vi "main_loop.vi"(8 "error in (no error)":errorcluster, 11 "control references":T2) -> (0 "error out":errorcluster)   [LabVIEW 2010]
uses:
  type_definitions/clusters/controls_refs.ctl
  type_definitions/enumerations/state_enumeration.ctl
  type_definitions/enumerations/main_trigger_enum.ctl
  type_definitions/clusters/state_data_cluster.ctl
  type_definitions/clusters/top_level_config_cluster.ctl
  common/clusters/plugin_specification.ctl
  common/enumerations/top-level_component_type_enum.ctl
  common/classes/GenericComponent/GenericComponent/GenericComponent.lvclass
  type_definitions/enumerations/main_control_types.ctl
  common/classes/NoteBook/Notebook/Notebook.lvclass
panel:
  out "state":T1
  out "Main statechart loop counter":i32
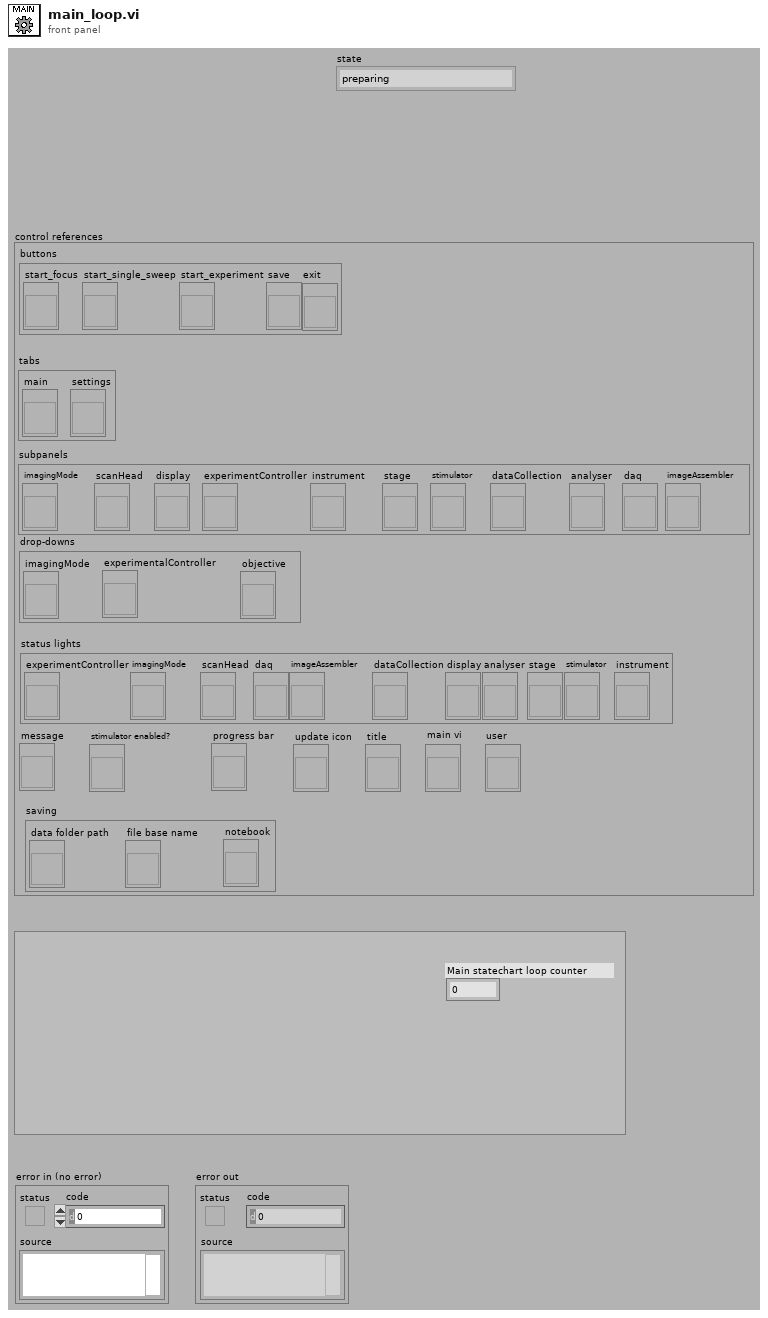
[diagram p1: front panel]
types:
  T1 = typedef "state_enumeration.ctl" = enum16{"preparing", "ready", "saving"}
  T2 = typedef "controls_refs.ctl" = cluster{"buttons":cluster{"start_focus":refnum<vi>, "start_single_sweep":refnum<vi>, "start_experiment":refnum<vi>, "save":refnum<vi>, "exit":refnum<vi>}, "tabs":cluster{"main":refnum<vi>, "settings":refnum<vi>}, "subpanels":cluster{"imagingMode":refnum<vi>, "scanHead":refnum<vi>, "display":refnum<vi>, "experimentController":refnum<vi>, "instrument":refnum<vi>, "stage":refnum<vi>, "stimulator":refnum<vi>, "dataCollection":refnum<vi>, "analyser":refnum<vi>, "daq":refnum<vi>, "imageAssembler":refnum<vi>}, "drop-downs":cluster{"imagingMode":refnum<vi>, "experimentalController":refnum<vi>, "objective":refnum<vi>}, "status lights":cluster{"experimentController":refnum<vi>, "imagingMode":refnum<vi>, "scanHead":refnum<vi>, "daq":refnum<vi>, "imageAssembler":refnum<vi>, "dataCollection":refnum<vi>, "display":refnum<vi>, "analyser":refnum<vi>, "stage":refnum<vi>, "stimulator":refnum<vi>, "instrument":refnum<vi>}, "message":refnum<vi>, "stimulator enabled?":refnum<vi>, "saving":cluster{"data folder path":refnum<vi>, "file base name":refnum<vi>, "notebook":refnum<vi>}, "progress bar":refnum<vi>, "update icon":refnum<vi>, "title":refnum<vi>, "main vi":refnum<vi>, "user":refnum<vi>}
  T3 = typedef "main_trigger_enum.ctl" = enum16{"NULL", "initialise", "terminate", "start", "stop", "change objective", "change experimentController", "change imagingMode", "save notebook", "started saving", "finished saving", "expCtr ready", "expCtr missing", "imgMd ready", "imgMd missing", "scanHd ready", "scanHd missing", "DAQ ready", "DAQ missing", "imgAsm ready", "imgAsm missing", "dataColl ready", "dataColl missing", "display ready", "display missing", "analysr ready", "analysr missing", "instrmnt ready", "instrmnt missing", "stimltr ready", "stimltr missing", "stage ready", "stage missing"}
  T4 = typedef "state_data_cluster.ctl" = cluster{"configuration":T5, "previous message display parameters":cluster{"previous  string":string, "BG slider":u32, "previously visible?":bool}}
  T5 = typedef "top_level_config_cluster.ctl" = cluster{"experimentControllers":T6[], "default experimentController":string, "imagingModes":T6[], "default imagingMode":string, "stage":T6, "objectives":T6[], "default objective":string}
  T6 = typedef "plugin_specification.ctl" = cluster{"class path":string, "configuration":string, "label":string, "settings name":string}
  T7 = typedef "top-level_component_type_enum.ctl" = enum16{"undefined", "ImagingMode", "ScanHead", "DAQ", "ImageAssembler", "Display", "DataCollection", "Analyser", "Stimulator", "ExperimentController", "Instrument", "Stage"}
  T8 = enum8{"Enabled", "Disabled", "Disabled and Grayed Out"}
  T9 = cluster{"previous  string":string, "BG slider":u32, "previously visible?":bool}
  T10 = typedef "main_control_types.ctl" = enum16{"scan start button", "experimentController subpanel", "imagingMode subpanel", "scanHead subpanel", "dataCollection subpanel", "display subpanel", "analyser subpanel", "stimulator subpanel", "imagingMode drop-down", "experimentController drop-down", "objective drop-down", "exit button"}
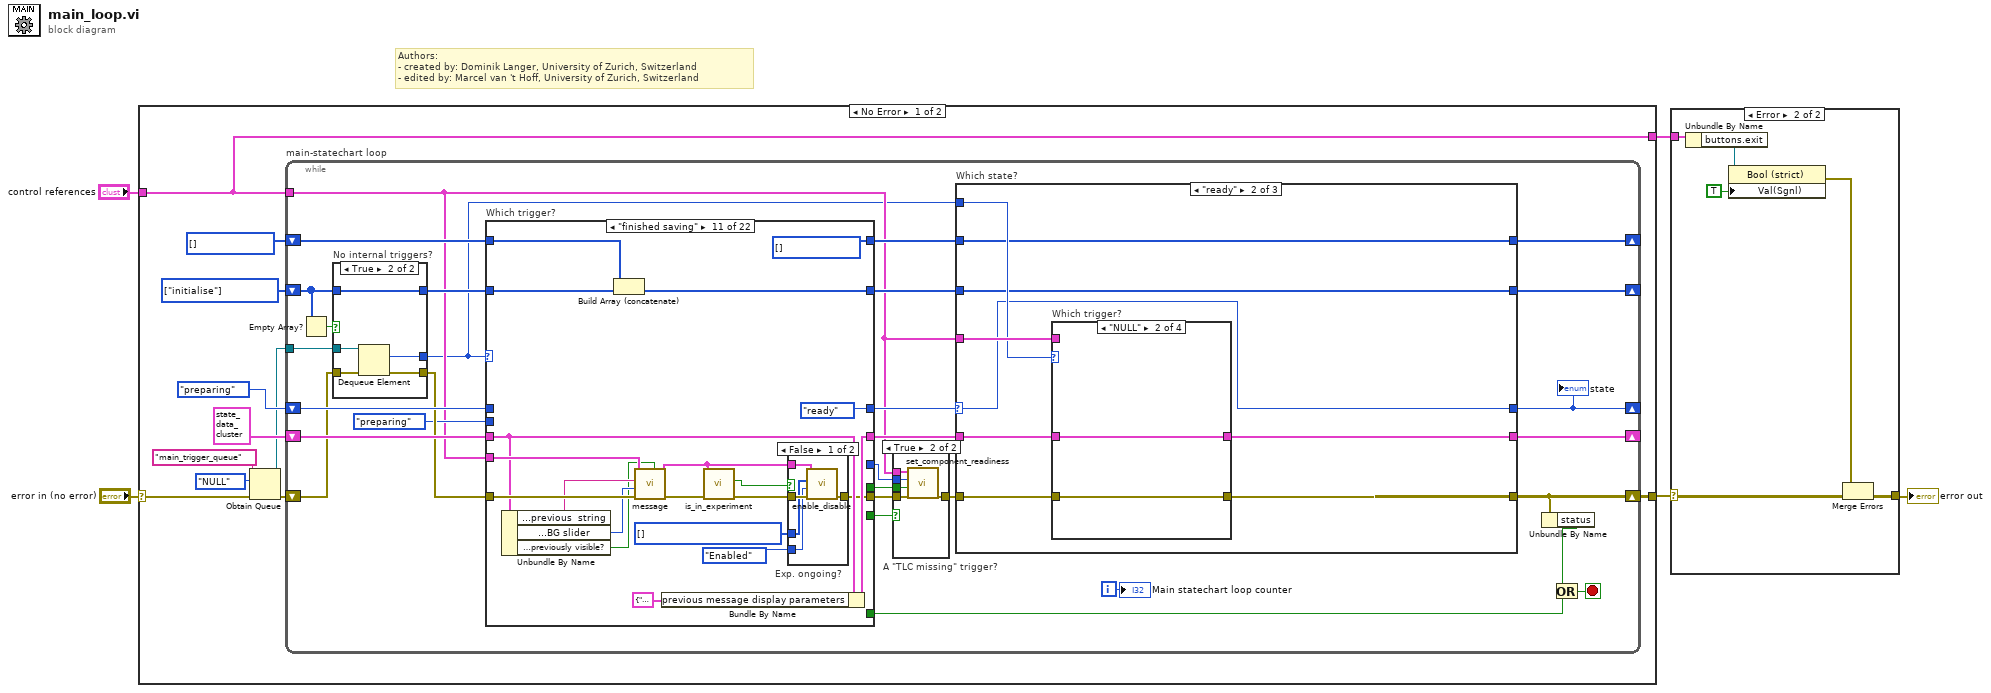
[diagram p0: block diagram]
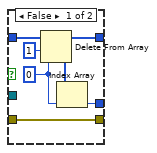
[diagram p3: hidden frame]
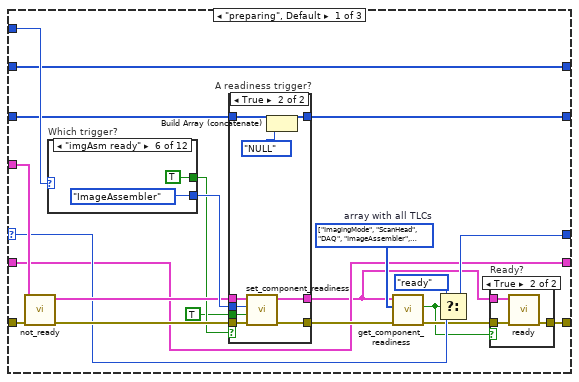
[diagram p5: hidden frame]
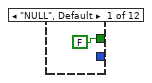
[diagram p8: hidden frame]
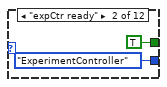
[diagram p9: hidden frame]
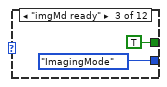
[diagram p10: hidden frame]
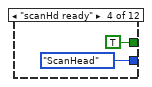
[diagram p11: hidden frame]
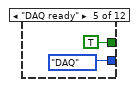
[diagram p12: hidden frame]
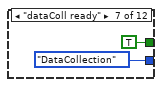
[diagram p13: hidden frame]
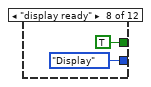
[diagram p14: hidden frame]
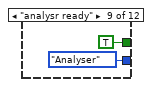
[diagram p15: hidden frame]
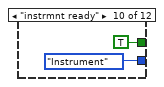
[diagram p16: hidden frame]
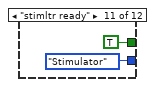
[diagram p17: hidden frame]
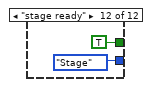
[diagram p18: hidden frame]
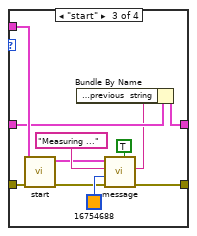
[diagram p20: hidden frame]
diagram:
  # "Authors: \n- created by: Dominik Langer, University of Zurich, Switzerland\n- edited by: Marcel van 't Hoff, University of Zurich, Switzerland"
  n1 = case shown="No Error" "error in (no error)" {
    selector: "error in (no error)" -> [w11 w376]
    tunnel: [w16 w376] -> w3
    tunnel: "control references" -> [w15 w375]
    tunnel: [w15 w375] -> w1
    frame No Error {
      w6 = T3[] [] items=["NULL", "initialise", "terminate", "start", "stop", "change objective", "change experimentController", "change imagingMode", "save notebook", "started saving", "finished saving", "expCtr ready", "expCtr missing", "imgMd ready", "imgMd missing", "scanHd ready", "scanHd missing", "DAQ ready", "DAQ missing", "imgAsm ready", "imgAsm missing", "dataColl ready", "dataColl missing", "display ready", "display missing", "analysr ready", "analysr missing", "instrmnt ready", "instrmnt missing", "stimltr ready", "stimltr missing", "stage ready", "stage missing"]
      w12 = T3[] [enum."initialise"] items=["NULL", "initialise", "terminate", "start", "stop", "change objective", "change experimentController", "change imagingMode", "save notebook", "started saving", "finished saving", "expCtr ready", "expCtr missing", "imgMd ready", "imgMd missing", "scanHd ready", "scanHd missing", "DAQ ready", "DAQ missing", "imgAsm ready", "imgAsm missing", "dataColl ready", "dataColl missing", "display ready", "display missing", "analysr ready", "analysr missing", "instrmnt ready", "instrmnt missing", "stimltr ready", "stimltr missing", "stage ready", "stage missing"]
      n2 = Obtain Queue(name (unnamed)="main_trigger_queue", element data type=main_trigger_enum."NULL" ("main trigger"), error in (no error)=w11) -> (queue out=w7:refnum<queue>, error out=w10:errorcluster)  [unwired: 2 in, 1 out]
      n3 = while "main-statechart loop" {
        tunnel: w15 -> [w19]
        shift-right: [w36] -> w16
        shift-left: w10 -> [w27]
        shift-right: [w37] -> _
        shift-left: T4 {"configuration"={"experimentControllers"=[], "default experimentController"="", "imagingModes"=[], "default imagingMode"="", "stage"={"class path"="", "configuration"="", "label"="", "settings name"=""}, "objectives"=[], "default objective"=""}, "previous message display parameters"={"previous  string"="", "BG slider"=16754688, "previously visible?"=FALSE}} ("state data") -> [w42]
        shift-right: [w39] -> _
        shift-left: state_enumeration."preparing" ("state enumeration") -> [w41]
        shift-right: [w35] -> _
        shift-left: w12 -> [w30]
        tunnel: w7 -> [w28]
        shift-right: [w24] -> _
        shift-left: w6 -> [w21]
        i -> [w46]
        stop <- w45 stop-if-true
        n4 = Empty Array?(array=w30) -> (empty?=w29:bool)
        n5 = case "No internal triggers?" shown="True" w29 {
          tunnel: w30 -> [w53 w58]
          tunnel: [w52 w58] -> w23
          tunnel: [w48 w56] -> w18
          tunnel: w28 -> [_ w57]
          tunnel: w27 -> [w47 w55]
          tunnel: [w47 w54] -> w26
          frame False {
            w49 = 0 ("index")
            n6 = Delete From Array(array=w53, length=1, index=w49) -> (deleted portion=w51:T3[], array with subset deleted=w52:T3[])
            n7 = Index Array(array=w51, index=w49) -> (element=w48:T3)
          }
          frame True {
            n8 = Dequeue Element(queue=w57, error in (no error)=w55) -> (element=w56:T3, error out=w54:errorcluster)  [unwired: 1 in, 2 out]
          }
        }
        n9 = case "Which trigger?" shown="\"finished saving\"" w18 {
          tunnel: w26 -> [w176 w185 w191 w202 w207 w216 w224 w233 w239 w246 w289 w303 w311 w318 w325 w332 w339 w346 w353 w360 w367 w374]
          tunnel: w19 -> [_ w186 w193 _ _ w214 w220 w231 _ w244 w288 _ _ _ _ _ _ _ _ _ _ _]
          tunnel: [w176 w184 w194 w202 w207 w215 w223 w232 w238 w258 w281 w303 w311 w318 w325 w332 w339 w346 w353 w360 w367 w374] -> w33
          tunnel: [_ _ TRUE _ _ _ _ _ _ _ _ _ _ _ _ _ _ _ _ _ _ _] -> w44
          tunnel: w42 -> [w177 w183 w196 w201 w206 w212 w221 w229 w237 w251 w283 w304 w310 w317 w324 w331 w338 w345 w352 w359 w366 w373]
          tunnel: [w177 w181 w196 w201 w206 w212 w221 w229 w237 w255 w282 w304 w310 w317 w324 w331 w338 w345 w352 w359 w366 w373] -> w38
          tunnel: w41 -> [w175 w180 _ w200 w205 w210 w219 w227 w236 _ _ _ _ _ _ _ _ _ _ _ _ _]
          tunnel: [w175 w180 state_enumeration."preparing" ("state enumeration") w200 w205 w210 w219 w227 w236 state_enumeration."saving" ("state enumeration") state_enumeration."ready" ("state enumeration") w299 w307 w314 w321 w328 w335 w342 w349 w356 w363 w370] -> w40
          tunnel: [_ _ _ _ _ _ _ _ _ _ _ top-level_component_type_enum."ExperimentController" ("top-level component type") top-level_component_type_enum."ImagingMode" ("top-level component type") top-level_component_type_enum."ScanHead" ("top-level component type") top-level_component_type_enum."DAQ" ("top-level component type") top-level_component_type_enum."ImageAssembler" ("top-level component type") top-level_component_type_enum."DataCollection" ("top-level component type") top-level_component_type_enum."Display" ("top-level component type") top-level_component_type_enum."Analyser" ("top-level component type") top-level_component_type_enum."Instrument" ("top-level component type") top-level_component_type_enum."Stimulator" ("top-level component type") top-level_component_type_enum."Stage" ("top-level component type")] -> w17
          tunnel: [_ _ _ _ _ _ _ _ _ _ _ FALSE _ _ _ _ _ _ _ _ _ _] -> w32
          tunnel: [_ _ _ _ _ _ _ _ _ _ _ TRUE TRUE TRUE TRUE TRUE TRUE TRUE TRUE TRUE TRUE TRUE] -> w31
          tunnel: state_enumeration."preparing" ("state enumeration") -> [_ _ _ _ _ _ _ _ _ _ _ w299 w307 w314 w321 w328 w335 w342 w349 w356 w363 w370]
          tunnel: w21 -> [w174 w179 w188 w199 w204 w209 w218 w226 w235 w248 w278 w298 w306 w313 w320 w327 w334 w341 w348 w355 w362 w369]
          tunnel: w23 -> [w173 w178 w187 w198 w203 w208 w217 w225 w234 w247 w277 w297 w305 w312 w319 w326 w333 w340 w347 w354 w361 w368]
          tunnel: [w173 w178 w187 w198 w203 w208 w217 w225 w234 w247 w276 w297 w305 w312 w319 w326 w333 w340 w347 w354 w361 w368] -> w22
          tunnel: [w174 w179 w188 w199 w204 w209 w218 w226 w235 w248 w275 w298 w306 w313 w320 w327 w334 w341 w348 w355 w362 w369] -> w20
          frame "NULL", Default {
          }
          frame "initialise" {
            n10 = call "initialise_main.vi"("error in (no error)"=w185, "control references in"=w186) -> ("error out"=w184:errorcluster, "configuration"=w182:T5)  [unwired: 8 in]
            n11 = Bundle By Name(cluster=w183, "configuration"=w182) -> (w181:T4)
          }
          frame "terminate" {
            n12 = Unbundle By Name(w193) -> ("buttons.exit"=w192:refnum<vi>)
            n13 = property class="Bool (strict)"(reference=w192, error in=w191, "Val(Sgnl)"=TRUE ("Value (Signaling)")) -> (error out=w190:errorcluster)  [unwired: 1 out]
            n14 = call "terminate_main.vi"("error in (no error)"=w190) -> ("error out"=w194:errorcluster)  [unwired: 10 in]
          }
          frame "start" {
          }
          frame "stop" {
          }
          frame "change objective" {
            n15 = Unbundle By Name(w212) -> ("configuration.objectives"=w211:T6[])
            n16 = Unbundle By Name(w214) -> ("drop-downs.objective"=w213:refnum<vi>)
            n17 = call "change_objective.vi"("error in (no error)"=w216, "objectives"=w211, "objective"=w213) -> ("error out"=w215:errorcluster)  [unwired: 8 in]
          }
          frame "change experimentController" {
            n18 = Unbundle By Name(w221) -> ("configuration.experimentControllers"=w222:T6[])
            n19 = call "change_experimentController.vi"("error in (no error)"=w224, "experimentControllers"=w222, "control references in"=w220) -> ("error out"=w223:errorcluster)  [unwired: 8 in]
          }
          frame "change imagingMode" {
            n20 = Unbundle By Name(w229) -> ("configuration.imagingModes"=w228:T6[])
            n21 = Unbundle By Name(w231) -> ("drop-downs.imagingMode"=w230:refnum<vi>)
            n22 = call "change_imagingMode.vi"("error in (no error)"=w233, "imagingModes"=w228, "imagingMode"=w230) -> ("error out"=w232:errorcluster)  [unwired: 8 in]
          }
          frame "save notebook" {
            n23 = call-dynamic "get_notebook.vi"("error in (no error)"=w239, "GenericComponent in"=refnum<class "GenericComponent.lvclass"> refnum) -> ("error out"=w240:errorcluster, "notebook"=w241:refnum<class "Notebook.lvclass">)  [unwired: 7 in, 1 out]
            n24 = call "save.vi"("error in (no error)"=w240, "Notebook in"=w241) -> ("error out"=w238:errorcluster)  [unwired: 8 in, 1 out]
          }
          frame "started saving" {
            w256 = T10[] [] items=["scan start button", "experimentController subpanel", "imagingMode subpanel", "scanHead subpanel", "dataCollection subpanel", "display subpanel", "analyser subpanel", "stimulator subpanel", "imagingMode drop-down", "experimentController drop-down", "objective drop-down", "exit button"] ("controls")
            n25 = call "is_in_experiment.vi"("error in (no error)"=w246, "control references"=w244) -> ("error out"=w245:errorcluster, "in experiment?"=w243:bool)  [unwired: 8 in]
            n26 = case "Experiment ongoing?" shown="False" w243 {
              tunnel: w245 -> [w268 w270]
              tunnel: [w267 w270] -> w261
              tunnel: w244 -> [w266 w269]
              tunnel: T8."Disabled and Grayed Out" ("state") -> [w265 _]
              tunnel: w256 -> [w264 _]
              tunnel: [w263 w269] -> w250
              frame False {
                n27 = call "enable_disable.vi"("error in (no error)"=w268, "state"=w265, "controls"=w264, "control references in"=w266) -> ("error out"=w267:errorcluster, "control references out"=w263:T2)  [unwired: 6 in]
              }
              frame True {
              }
            }
            n28 = call "message.vi"("visible?"=TRUE, "error in (no error)"=w261, "BG slider"=u32 16751378, "text"="Saving ...", "control references in"=w250) -> ("error out"=w258:errorcluster, "previous text"=w254:string, "previously visible?"=w252:bool, "previous BG colour"=w253:u32)  [unwired: 2 in, 1 out]
            n29 = Bundle By Name(cluster=w251, "previous message display parameters.previous  string"=w254, "previous message display parameters.BG slider"=w253, "previous message display parameters.previously visible?"=w252) -> (w255:T4)
          }
          frame "finished saving" {
            w275 = T3[] [] items=["NULL", "initialise", "terminate", "start", "stop", "change objective", "change experimentController", "change imagingMode", "save notebook", "started saving", "finished saving", "expCtr ready", "expCtr missing", "imgMd ready", "imgMd missing", "scanHd ready", "scanHd missing", "DAQ ready", "DAQ missing", "imgAsm ready", "imgAsm missing", "dataColl ready", "dataColl missing", "display ready", "display missing", "analysr ready", "analysr missing", "instrmnt ready", "instrmnt missing", "stimltr ready", "stimltr missing", "stage ready", "stage missing"]
            w280 = T10[] [] items=["scan start button", "experimentController subpanel", "imagingMode subpanel", "scanHead subpanel", "dataCollection subpanel", "display subpanel", "analyser subpanel", "stimulator subpanel", "imagingMode drop-down", "experimentController drop-down", "objective drop-down", "exit button"] ("controls")
            n30 = Unbundle By Name(w283) -> ("previous message display parameters.previous  string"=w287:string, "previous message display parameters.BG slider"=w286:u32, "previous message display parameters.previously visible?"=w285:bool)
            n31 = Build Array (concatenate)(w278, w277) -> (w276:T3[])
            n32 = call "message.vi"("visible?"=w285, "error in (no error)"=w289, "BG slider"=w286, "text"=w287, "control references in"=w288) -> ("error out"=w274:errorcluster, "control references out"=w271:T2)  [unwired: 2 in, 3 out]
            n33 = Bundle By Name(cluster=w283, "previous message display parameters"=T9 {"previous  string"="", "BG slider"=0, "previously visible?"=FALSE}) -> (w282:T4)
            n34 = call "is_in_experiment.vi"("error in (no error)"=w274, "control references"=w271) -> ("error out"=w273:errorcluster, "in experiment?"=w272:bool)  [unwired: 8 in]
            n35 = case "Exp. ongoing?" shown="False" w272 {
              tunnel: w273 -> [w295 w296]
              tunnel: [w294 w296] -> w281
              tunnel: w271 -> [w293 _]
              tunnel: w280 -> [w292 _]
              tunnel: T8."Enabled" ("state") -> [w291 _]
              frame False {
                n36 = call "enable_disable.vi"("error in (no error)"=w295, "state"=w291, "controls"=w292, "control references in"=w293) -> ("error out"=w294:errorcluster)  [unwired: 6 in, 1 out]
              }
              frame True {
              }
            }
          }
          frame "expCtr missing" {
          }
          frame "imgMd missing" {
          }
          frame "scanHd missing" {
          }
          frame "DAQ missing" {
          }
          frame "imgAsm missing" {
          }
          frame "dataColl missing" {
          }
          frame "display missing" {
          }
          frame "analysr missing" {
          }
          frame "instrmnt missing" {
          }
          frame "stimltr missing" {
          }
          frame "stage missing" {
          }
        }
        n37 = case "A \"TLC missing\" trigger?" shown="True" w31 {
          tunnel: [w59 w64] -> w34
          tunnel: w33 -> [w59 w63]
          tunnel: w19 -> [_ w62]
          tunnel: w17 -> [_ w61]
          tunnel: w32 -> [_ w60]
          frame False {
          }
          frame True {
            n38 = call "set_component_readiness.vi"("error in (no error)"=w63, "ready?"=w60, "top-level component type"=w61, "control references in"=w62) -> ("error out"=w64:errorcluster)  [unwired: 6 in, 1 out]
          }
        }
        n39 = case "Which state?" shown="\"ready\"" w40 {
          selector: w40 -> [w74 w126 w168]
          tunnel: w34 -> [w81 w132 w166]
          tunnel: [w76 w126 w168] -> w39
          tunnel: w38 -> [w70 w130 w167]
          tunnel: [w70 w129 w167] -> w37
          tunnel: [w67 w128 w166] -> w36
          tunnel: w18 -> [w78 w131 w162]
          tunnel: w19 -> [w82 w133 _]
          tunnel: w22 -> [w72 w127 w165]
          tunnel: [w71 w127 w165] -> w35
          tunnel: w20 -> [w69 w125 w164]
          tunnel: [w69 w125 w163] -> w24
          frame "preparing", Default {
            w80 = T7[] [enum."ImagingMode", enum."ScanHead", enum."DAQ", enum."ImageAssembler", enum."Display", enum."DataCollection", enum."Analyser", enum."Stimulator", enum."ExperimentController", enum."Instrument", enum."Stage"] items=["undefined", "ImagingMode", "ScanHead", "DAQ", "ImageAssembler", "Display", "DataCollection", "Analyser", "Stimulator", "ExperimentController", "Instrument", "Stage"]  # array with all TLCs
            n40 = call "not_ready.vi"("error in (no error)"=w81, "control references in"=w82) -> ("error out"=w85:errorcluster, "control references out"=w83:T2)  [unwired: 8 in]
            n41 = case "Which trigger?" shown="\"imgAsm ready\"" w78 {
              tunnel: [_ top-level_component_type_enum."ExperimentController" ("top-level component type") top-level_component_type_enum."ImagingMode" ("top-level component type") top-level_component_type_enum."ScanHead" ("top-level component type") top-level_component_type_enum."DAQ" ("top-level component type") top-level_component_type_enum."ImageAssembler" ("top-level component type") top-level_component_type_enum."DataCollection" ("top-level component type") top-level_component_type_enum."Display" ("top-level component type") top-level_component_type_enum."Analyser" ("top-level component type") top-level_component_type_enum."Instrument" ("top-level component type") top-level_component_type_enum."Stimulator" ("top-level component type") top-level_component_type_enum."Stage" ("top-level component type")] -> w84
              tunnel: [FALSE TRUE TRUE TRUE TRUE TRUE TRUE TRUE TRUE TRUE TRUE TRUE] -> w77
              frame "NULL", Default {
              }
              frame "expCtr ready" {
              }
              frame "imgMd ready" {
              }
              frame "scanHd ready" {
              }
              frame "DAQ ready" {
              }
              frame "imgAsm ready" {
              }
              frame "dataColl ready" {
              }
              frame "display ready" {
              }
              frame "analysr ready" {
              }
              frame "instrmnt ready" {
              }
              frame "stimltr ready" {
              }
              frame "stage ready" {
              }
            }
            n42 = case "A readiness trigger?" shown="True" w77 {
              tunnel: w85 -> [w92 w101]
              tunnel: w84 -> [_ w100]
              tunnel: TRUE -> [_ w99]
              tunnel: w83 -> [w91 w98]
              tunnel: [w92 w97] -> w79
              tunnel: [w91 w96] -> w66
              tunnel: w72 -> [w90 w95]
              tunnel: [w90 w93] -> w71
              frame False {
              }
              frame True {
                n43 = call "set_component_readiness.vi"("error in (no error)"=w101, "ready?"=w99, "top-level component type"=w100, "control references in"=w98) -> ("error out"=w97:errorcluster, "control references out"=w96:T2)  [unwired: 6 in]
                n44 = Build Array (concatenate)(w95, main_trigger_enum."NULL" ("main trigger")) -> (w93:T3[])
              }
            }
            n45 = call "get_component_readiness.vi"("error in (no error)"=w79, "top-level components"=w80, "control references"=w66) -> ("error out"=w68:errorcluster, "ready?"=w65:bool)  [unwired: 7 in]
            n46 = Select(t=state_enumeration."ready" ("state enumeration"), s=w65, f=w74) -> (s? t:f=w76:T1)
            n47 = case "Ready?" shown="True" w65 {
              tunnel: w68 -> [w86 w89]
              tunnel: [w86 w88] -> w67
              tunnel: w66 -> [_ w87]
              frame False {
              }
              frame True {
                n48 = call "ready.vi"("error in (no error)"=w89, "control refs in"=w87) -> ("error out"=w88:errorcluster)  [unwired: 8 in, 1 out]
              }
            }
          }
          frame "ready" {
            n49 = case "Which trigger?" shown="\"NULL\"" w131 {
              tunnel: w133 -> [_ _ w143 w154]
              tunnel: w132 -> [w134 w136 w142 w153]
              tunnel: w130 -> [w135 w137 w141 w150]
              tunnel: [w135 w137 w140 w149] -> w129
              tunnel: [w134 w136 w138 w152] -> w128
              frame Default {
              }
              frame "NULL" {
              }
              frame "start" {
                n50 = call "start.vi"("error in (no error)"=w142, "control references in"=w143) -> ("error out"=w145:errorcluster, "control references out"=w146:T2)  [unwired: 8 in]
                n51 = call "message.vi"("visible?"=TRUE, "error in (no error)"=w145, "BG slider"=u32 16754688, "text"="Measuring ...", "control references in"=w146) -> ("error out"=w138:errorcluster, "previous text"=w139:string)  [unwired: 2 in, 3 out]
                n52 = Bundle By Name(cluster=w141, "previous message display parameters.previous  string"=w139) -> (w140:T4)
              }
              frame "stop" {
                n53 = call "stop.vi"("error in (no error)"=w153, "control references in"=w154) -> ("error out"=w158:errorcluster, "control references out"=w157:T2)  [unwired: 8 in]
                n54 = call "message.vi"("visible?"=TRUE, "error in (no error)"=w158, "BG slider"=u32 4499968, "text"="READY", "control references in"=w157) -> ("error out"=w152:errorcluster, "previous text"=w151:string)  [unwired: 2 in, 3 out]
                n55 = Bundle By Name(cluster=w150, "previous message display parameters.previous  string"=w151) -> (w149:T4)
              }
            }
          }
          frame "saving" {
            n56 = Not Equal?(x=w162, y=main_trigger_enum."started saving") -> (x != y?=w160:bool)
            n57 = case "Keep trigger for later?" shown="True" w160 {
              tunnel: w164 -> [w169 w172]
              tunnel: [w169 w171] -> w163
              tunnel: w162 -> [_ w170]
              frame False {
              }
              frame True {
                n58 = Build Array (concatenate)(w172, w170) -> (w171:T3[])
              }
            }
          }
        }
        "state" <- w39
        n59 = Unbundle By Name(w36) -> ("status"=w43:bool)
        n60 = Or(x=w43, y=w44) -> (x .or. y?=w45:bool)
        "Main statechart loop counter" <- w46
      }
    }
    frame Error {
    }
  }
  n61 = case shown="Error" w3 {
    selector: w3 -> [w377 w383]
    tunnel: [w377 w382] -> w2
    tunnel: w1 -> [_ w379]
    frame No Error {
    }
    frame Error {
      n62 = Unbundle By Name(w379) -> ("buttons.exit"=w381:refnum<vi>)
      n63 = property class="Bool (strict)"(reference=w381, "Val(Sgnl)"=TRUE ("Value (Signaling)")) -> (error out=w378:errorcluster)  [unwired: 1 in, 1 out]
      n64 = Merge Errors(w378, w383) -> (w382:errorcluster)
    }
  }
  "error out" <- w2
